vi "create html.vi"(8 "error in (no error)":errorcluster caption="错误输入（无错误）", 10 "data":string[][](array[string]), 11 "columns":string[](array[string])) -> (0 "error out":errorcluster caption="错误输出", 3 "url":string)   [LabVIEW 2016, in "数据查询.lvlib"]
panel:
  out "结果字符串":string
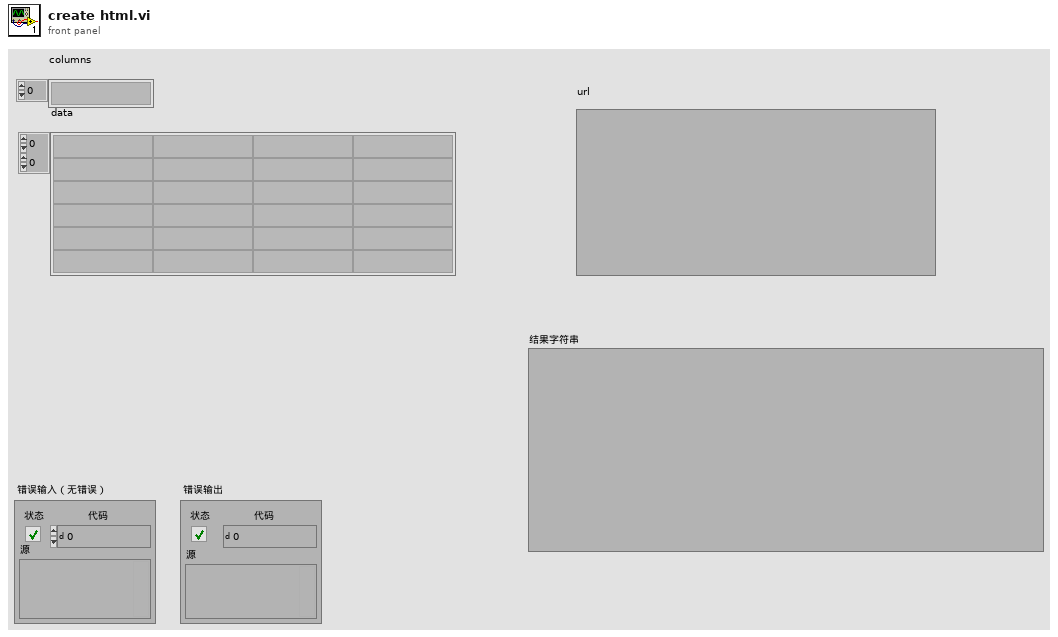
[diagram p1: front panel]
types:
  T1 = enum16{"open", "replace", "create", "open or create", "replace or create", "replace or create with confirmation"}
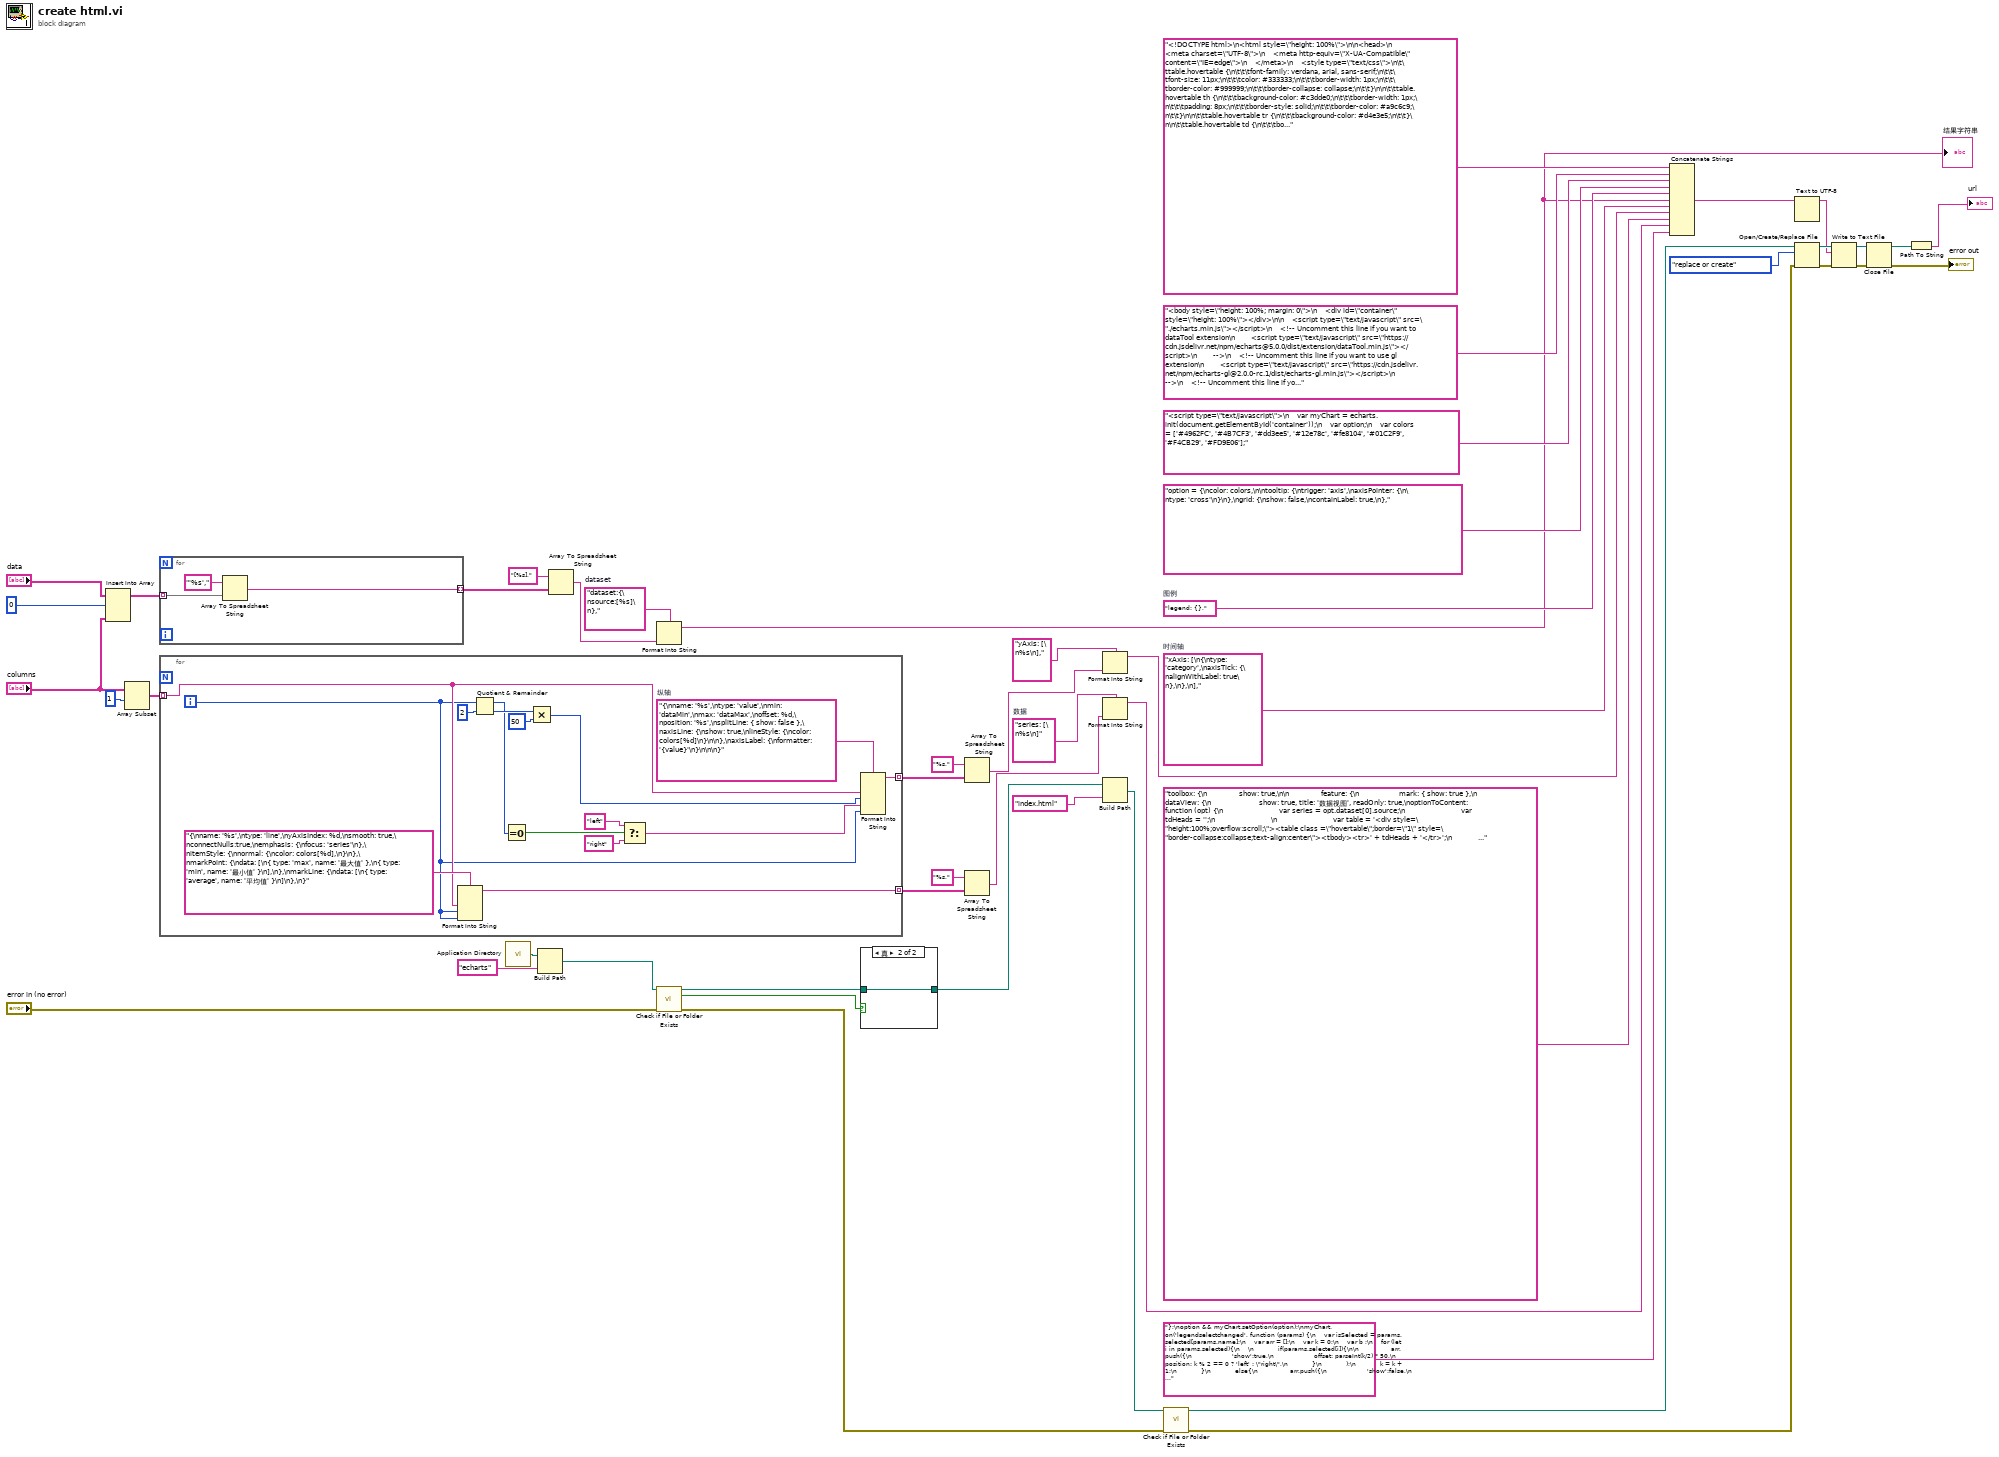
[diagram p0: block diagram]
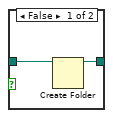
[diagram p2: hidden frame]
diagram:
  w13 = "dataset:{\nsource:[%s]\n},"  # dataset
  w44 = "series: [\n%s\n]"  # 数据
  w9 = "xAxis: [\n{\ntype: 'category',\naxisTick: {\nalignWithLabel: true\n},\n},\n],"  # 时间轴
  w10 = "legend: {},"  # 图例
  n1 = Insert Into Array(array="data", index (row)=0 ("索引 (行)"), new element="columns") -> (w6:string[][])  [unwired: 1 in]
  n2 = Array Subset(array="columns", index=1 ("索引")) -> (w1:string[])  [unwired: 1 in]
  n3 = for {
    tunnel: w6 -> [w54] mode=indexing
    tunnel: [w52] -> w11 mode=indexing
    n4 = Array To Spreadsheet String(array=w54, 3:"'%s'," ("格式字符串")) -> (spreadsheet string=w52:string)  [unwired: 1 in]
  }
  n5 = for {
    tunnel: w1 -> [w64] mode=indexing
    tunnel: [w68] -> w40 mode=indexing
    tunnel: [w66] -> w37 mode=indexing
    i -> [w55]
    w69 = "{\nname: '%s',\ntype: 'value',\nmin: 'dataMin',\nmax: 'dataMax',\noffset: %d,\nposition: '%s',\nsplitLine: { show: false },\naxisLine: {\nshow: true,\nlineStyle: {\ncolor: colors[%d]\n}\n\n},\naxisLabel: {\nformatter: '{value}'\n}\n\n\n}"  # 纵轴
    n6 = Format Into String(format string="{\nname: '%s',\ntype: 'line',\nyAxisIndex: %d,\nsmooth: true,\nconnectNulls:true,\nemphasis: {\nfocus: 'series'\n},\nitemStyle: {\nnormal: {\ncolor: colors[%d],\n}\n},\nmarkPoint: {\ndata: [\n{ type: 'max', name: '最大值' },\n{ type: 'min', name: '最小值' }\n],\n},\nmarkLine: {\ndata: [\n{ type: 'average', name: '平均值' }\n]\n},\n}", w64, w55, w55) -> (resulting string=w66:string)  [unwired: 2 in, 1 out]
    n7 = Quotient & Remainder(x=w55, y=2) -> (x-y*floor(x/y)=w60:i32, floor(x/y)=w63:i32)
    n8 = Equal To 0?(x=w60) -> (x = 0?=w59:bool)
    n9 = Multiply(x=w63, y=50) -> (x*y=w61:i32)
    n10 = Select(t="left", s=w59, f="right") -> (s? t:f=w56:string)
    n11 = Format Into String(format string=w69, w64, w61, w56, w55) -> (resulting string=w68:string)  [unwired: 2 in, 1 out]
  }
  n12 = call <vilib>:"Application Directory.vi"() -> ("Application Directory"=w35:path)
  n13 = Build Path(base path=w35, name or relative path="echarts" ("名称或相对路径")) -> (appended path=w33:path)
  n14 = Array To Spreadsheet String(array=w11, 3:"[%s]," ("格式字符串")) -> (spreadsheet string=w8:string)  [unwired: 1 in]
  n15 = Format Into String(format string=w13, w8) -> (resulting string=w7:string)  [unwired: 2 in, 1 out]
  "结果字符串" <- w7
  n16 = call <vilib>:"Check if File or Folder Exists.vi"("error in (no error)"="error in (no error)", "path"=w33) -> ("error out"=w25:errorcluster, "file or folder exists?"=w32:bool, "dup path"=w31:path)  [unwired: 7 in]
  n17 = case shown="真" w32 {
    tunnel: w31 -> [w71 w72]
    tunnel: [w70 w72] -> w30
    frame False {
      n18 = Create Folder(path (use dialog)=w71) -> (created path=w70:path)  [unwired: 2 in, 2 out]
    }
    frame True {
    }
  }
  n19 = Array To Spreadsheet String(array=w40, 3:"%s," ("格式字符串")) -> (spreadsheet string=w39:string)  [unwired: 1 in]
  n20 = Array To Spreadsheet String(array=w37, 3:"%s," ("格式字符串")) -> (spreadsheet string=w36:string)  [unwired: 1 in]
  n21 = Format Into String(format string="yAxis: [\n%s\n],", w39) -> (resulting string=w46:string)  [unwired: 2 in, 1 out]
  n22 = Format Into String(format string=w44, w36) -> (resulting string=w43:string)  [unwired: 2 in, 1 out]
  n23 = Build Path(base path=w30, name or relative path="index.html" ("名称或相对路径")) -> (appended path=w28:path)
  n24 = call <vilib>:"Check if File or Folder Exists.vi"("error in (no error)"=w25, "path"=w28) -> ("error out"=w26:errorcluster, "dup path"=w27:path)  [unwired: 7 in, 1 out]
  n25 = Concatenate Strings("<!DOCTYPE html>\n<html style=\"height: 100%\">\n\n<head>\n    <meta charset=\"UTF-8\">\n    <meta http-equiv=\"X-UA-Compatible\" content=\"IE=edge\">\n    </meta>\n    <style type=\"text/css\">\n\t\ttable.hovertable {\n\t\t\tfont-family: verdana, arial, sans-serif;\n\t\t\tfont-size: 11px;\n\t\t\tcolor: #333333;\n\t\t\tborder-width: 1px;\n\t\t\tborder-color: #999999;\n\t\t\tborder-collapse: collapse;\n\t\t}\n\n\t\ttable.hovertable th {\n\t\t\tbackground-color: #c3dde0;\n\t\t\tborder-width: 1px;\n\t\t\tpadding: 8px;\n\t\t\tborder-style: solid;\n\t\t\tborder-color: #a9c6c9;\n\t\t}\n\n\t\ttable.hovertable tr {\n\t\t\tbackground-color: #d4e3e5;\n\t\t}\n\n\t\ttable.hovertable td {\n\t\t\tborder-width: 1px;\n\t\t\tpadding: 8px;\n\t\t\tborder-style: solid;\n\t\t\tborder-color: #a9c6c9;\n\t\t}\n\t</style>\n</head>", "<body style=\"height: 100%; margin: 0\">\n    <div id=\"container\" style=\"height: 100%\"></div>\n\n    <script type=\"text/javascript\" src=\"./echarts.min.js\"></script>\n    <!-- Uncomment this line if you want to dataTool extension\n        <script type=\"text/javascript\" src=\"https://cdn.jsdelivr.net/npm/echarts@5.0.0/dist/extension/dataTool.min.js\"></script>\n        -->\n    <!-- Uncomment this line if you want to use gl extension\n        <script type=\"text/javascript\" src=\"https://cdn.jsdelivr.net/npm/echarts-gl@2.0.0-rc.1/dist/echarts-gl.min.js\"></script>\n        -->\n    <!-- Uncomment this line if you want to echarts-stat extension\n        <script type=\"text/javascript\" src=\"https://cdn.jsdelivr.net/npm/echarts-stat@latest/dist/ecStat.min.js\"></script>\n        -->\n    <!-- Uncomment this line if you want to use map\n        <script type=\"text/javascript\" src=\"https://cdn.jsdelivr.net/npm/echarts@5.0.0/map/js/china.js\"></script>\n        <script type=\"text/javascript\" src=\"https://cdn.jsdelivr.net/npm/echarts@5.0.0/map/js/world.js\"></script>\n        -->\n    <!-- Uncomment these two lines if you want to use bmap extension\n        <script type=\"text/javascript\" src=\"https://api.map.baidu.com/api?v=2.0&ak=<Your Key Here>\"></script>\n        <script type=\"text/javascript\" src=\"https://cdn.jsdelivr.net/npm/echarts@5.0.0/dist/extension/bmap.min.js\"></script>\n        -->", "<script type=\"text/javascript\">\n    var myChart = echarts.init(document.getElementById('container'));\n    var option;\n    var colors = ['#4962FC', '#4B7CF3', '#dd3ee5', '#12e78c', '#fe8104', '#01C2F9', '#F4CB29', '#FD9E06'];", "option = {\ncolor: colors,\n\ntooltip: {\ntrigger: 'axis',\naxisPointer: {\n\ntype: 'cross'\n}\n},\ngrid: {\nshow: false,\ncontainLabel: true,\n},", w10, w7, w9, w46, "toolbox: {\n                show: true,\n\n                feature: {\n                    mark: { show: true },\n                    dataView: {\n                        show: true, title: '数据视图', readOnly: true,\noptionToContent: function (opt) {\n                            var series = opt.dataset[0].source;\n                            var tdHeads = '';\n                            \n                            var table = '<div style=\"height:100%;overflow:scroll;\"><table class =\"hovertable\";border=\"1\" style=\"border-collapse:collapse;text-align:center\"><tbody><tr>' + tdHeads + '</tr>';\n                            var tdBodys = '';\n                            for (var i = 0, l = series.length; i < l; i++) {\n                                for (var j = 0; j < series[0].length; j++) {\n                                    if (typeof (series[i][j]) == 'object') {\n\n \n                                        tdBodys += '<td>' + series[i][j] + '</td>';\n                                    } else {\n                                        tdBodys += '<td>' + series[i][j] + '</td>';\n                                    }\n                                }\n                                table += '<tr onmouseover=\"this.style.backgroundColor=&#39;#ffff66&#39;;\" onmouseout=\"this.style.backgroundColor=&#39;#d4e3e5&#39;;\" style=\"background-color: rgb(212, 227, 229);\">' + tdBodys + '</tr>';\n                                tdBodys = '';\n                            }\n                            table += '</tbody></table></div>';\n                            return table;\n                        }\n                    },\n                    magicType: { show: true, title: { line: '折线图', bar: '柱状图', }, type: ['line', 'bar'] },\n                    restore: { show: true, title: '刷新' },\n                    saveAsImage: { show: true, title: '保存图片', backgroundColor: '#fff' },\n                }\n            },\n\n\ndataZoom: [ { show: true, type: 'slider' , realtime: true, start: 0, end: 100, height: 50,\n                bottom: 10, }, { type: 'inside' , start: 0, end: 100 }, ],", w43, "};\noption && myChart.setOption(option);\nmyChart.on('legendselectchanged', function (params) {\n    var isSelected = params.selected[params.name];\n    var arr = [];\n    var k = 0;\n    var b ;\n    for (let i in params.selected){\n    \n            if(params.selected[i]){\n\n                arr.push({\n                    'show':true,\n                    offset: parseInt(k/2) * 50,\n                    position: k % 2 == 0 ? 'left' : \"right\",\n            }\n            );\n            k = k + 1;\n            }\n            else{\n                arr.push({\n                    'show':false,\n                    offset: 0,\n                });\n            }\n    };\nb = {yAxis:JSON.parse(JSON.stringify(arr))};\n    option && myChart.setOption(b);\n});\n</script>\n</body>\n\n</html>") -> (w15:string)
  n26 = Text to UTF-8(11:w15) -> (3:w14:string)  [unwired: 2 in, 1 out]
  n27 = Open/Create/Replace File(file path (use dialog)=w27, error in=w26, operation (0:open)=T1."replace or create" ("操作(0:open)")) -> (refnum out=w21:refnum<file>, error out=w22:errorcluster)  [unwired: 3 in, 1 out]
  n28 = Write to Text File(file (use dialog)=w21, text=w14, error in=w22) -> (refnum out=w20:refnum<file>, error out=w19:errorcluster)  [unwired: 1 in, 1 out]
  n29 = Close File(refnum=w20, error in=w19) -> (path=w18:path, error out=→"error out":errorcluster)
  n30 = Path To String(path=w18) -> (string=→"url":string)
